vi "Get_Target_Info.vi"(7 "Camera Orientation":cluster{"Yaw":dbl, "Elevation":dbl}, 8 "Height":T1, 9 "Target Location":cluster{"X (Pixels)":dbl, "Y (Pixels)":dbl}, 10 "Resolution":cluster{"H (pixels)":dbl, "V (Pixels)":dbl}, 11 "FOV":cluster{"X (degrees)":dbl, "Y (degrees)":dbl}) -> (0 "Distance (lateral)":dbl, 1 "Distance (CT)":dbl, 2 "Elevation Delta":dbl, 3 "Yaw Delta":dbl, 4 "Adjusted Elevation Delta":dbl, 5 "Adjusted Yaw Delta":dbl)   [LabVIEW 2016]
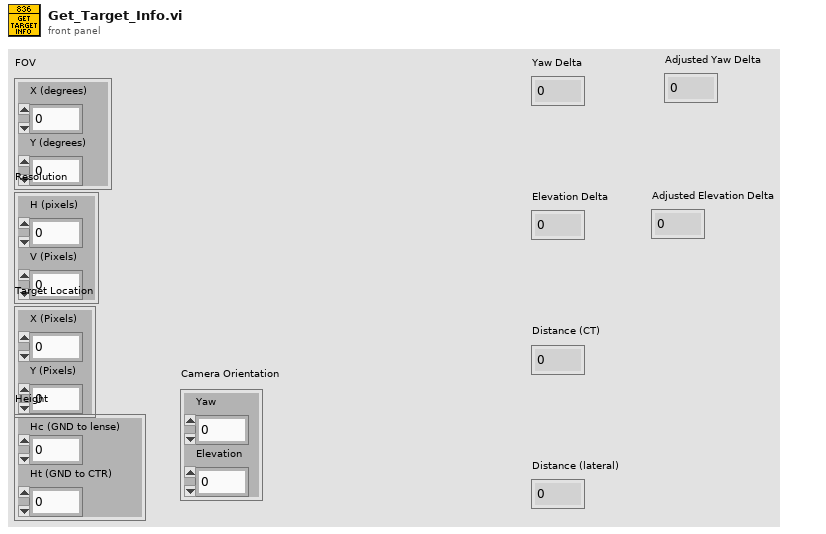
[diagram p1: front panel]
types:
  T1 = cluster{"Hc (GND to lense)":dbl, "Ht (GND to CTR)":dbl}
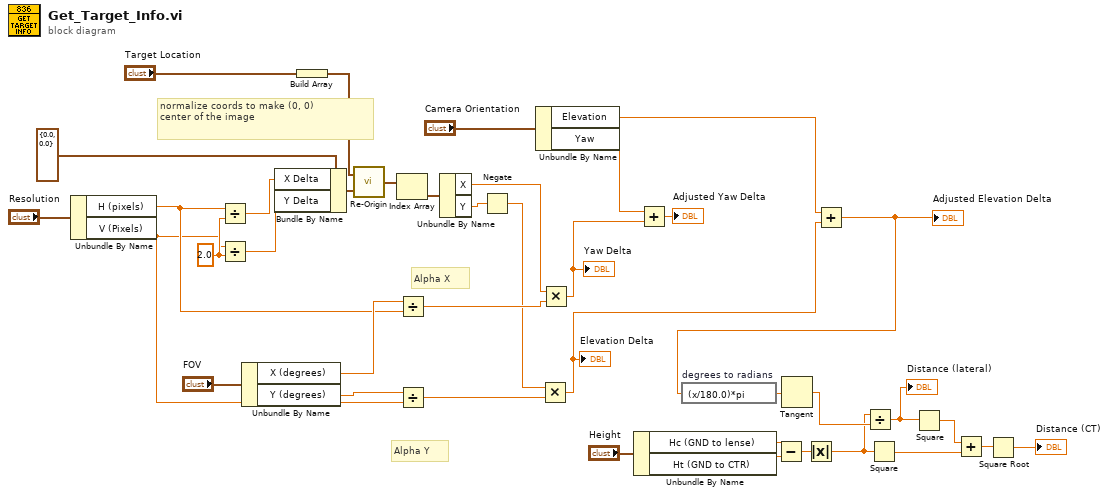
[diagram p0: block diagram]
diagram:
  w35 = 2.0 ("y")
  # "Alpha Y"
  # "Alpha X"
  # "normalize coords to make (0, 0)\ncenter of the image"
  n1 = Unbundle By Name("Resolution") -> ("H (pixels)"=w29:dbl, "V (Pixels)"=w24:dbl)
  n2 = Divide(x=w29, y=w35) -> (x/y=w34:dbl)
  n3 = Divide(x=w24, y=w35) -> (x/y=w33:dbl)
  n4 = Unbundle By Name("FOV") -> ("X (degrees)"=w30:dbl, "Y (degrees)"=w28:dbl)
  n5 = Bundle By Name(cluster=cluster{"X Delta":dbl, "Y Delta":dbl} {"X Delta"=0.0, "Y Delta"=0.0} ("Transition"), "X Delta"=w34, "Y Delta"=w33) -> (w32:cluster{"X Delta":dbl, "Y Delta":dbl})
  n6 = Build Array("Target Location") -> (w37:cluster{"X (Pixels)":dbl, "Y (Pixels)":dbl}[])
  n7 = call "Re-Origin.vi"("Transition"=w32, "Coordinates"=w37) -> ("Normalized Coords"=w26:cluster{"X":dbl, "Y":dbl}[])
  n8 = Index Array(array=w26) -> (element=w25:cluster{"X":dbl, "Y":dbl})  [unwired: 1 in]
  n9 = Divide(x=w30, y=w29) -> (x/y=w27:dbl)
  n10 = Divide(x=w28, y=w24) -> (x/y=w23:dbl)
  n11 = Unbundle By Name(w25) -> ("X"=w22:dbl, "Y"=w21:dbl)
  n12 = Negate(x=w21) -> (-x=w8:dbl)
  n13 = Unbundle By Name("Camera Orientation") -> ("Elevation"=w3:dbl, "Yaw"=w5:dbl)
  n14 = Multiply(x=w8, y=w23) -> (x*y=w2:dbl)
  "Elevation Delta" <- w2
  n15 = Multiply(x=w22, y=w27) -> (x*y=w6:dbl)
  "Yaw Delta" <- w6
  n16 = Unbundle By Name("Height") -> ("Hc (GND to lense)"=w19:dbl, "Ht (GND to CTR)"=w18:dbl)
  n17 = Add(x=w5, y=w6) -> (x+y=→"Adjusted Yaw Delta":dbl)
  n18 = Subtract(x=w19, y=w18) -> (x-y=w17:dbl)
  n19 = Absolute Value(x=w17) -> (abs(x)=w14:dbl)
  n20 = Add(x=w3, y=w2) -> (x+y=w1:dbl)
  "Adjusted Elevation Delta" <- w1
  n21 = expression code="(x/180.0)*pi" "degrees to radians"(w1) -> (w9:dbl)
  n22 = Tangent(1:w9) -> (0:w16:dbl)
  n23 = Divide(x=w14, y=w16) -> (x/y=w15:dbl)
  "Distance (lateral)" <- w15
  n24 = Square(x=w14) -> (x^2=w12:dbl)
  n25 = Square(x=w15) -> (x^2=w13:dbl)
  n26 = Add(x=w13, y=w12) -> (x+y=w11:dbl)
  n27 = Square Root(x=w11) -> (sqrt(x)=→"Distance (CT)":dbl)
